vi "Replace -2 and -1.vi"(5 "Row  [ ] IN":T2, 9 "Table size":cluster{"# Column":u16, "# Row":u16}) -> (6 "Row  [ ] OUT":T2, 10 "Row and #colums [ ]":T1(array[cluster]))   [LabVIEW 2019, in "Exaprom PDF.lvlib"]
doc: "Version 1.1\nDeveloped by Jean-Marc Simard\nCopyright © 2012, Exaprom Inc.\nAll rights reserved.\nLicense: BSD\n\nWith iTextSharp 4.1.6 (http://itextsharp.sourceforge.net)\nunder Mozilla Public License Version 1.1\n(http://www.mozilla.org/MPL/MPL-1.1.html)"
uses:
  Controls/Table Controls/Table Appearance and Font Row [ ].ctl
  Controls/Table Controls/One Row Appearance.ctl
  Controls/Table Controls/Row from to.ctl
  Controls/Table Controls/Cell, Alignment, LS and Font - hide Vmerge.ctl
  Controls/Table Controls/Cell Type, Alignment and LS.ctl
  Controls/Table Controls/Cell Alignment 20px.ctl
  Controls/Table Controls/Text vertical arrangement.ctl
  Controls/Text Controls/Line spacing.ctl
  Controls/Table Controls/Cell Appearance.ctl
  Controls/Table Controls/Cell Border 20 px.ctl
  Controls/Table Controls/Merge Horizontal.ctl
  Controls/Table Controls/Merge Vertical.ctl
  Controls/Font Controls/Font complete cluster.ctl
  Controls/Font Controls/Font size.ctl
  Controls/Font Controls/Font color.ctl
  Controls/Font Controls/Type and encoding.ctl
  Controls/Text Controls/Unicode/Type and run direction.ctl
  Exaprom PDF.lvlib
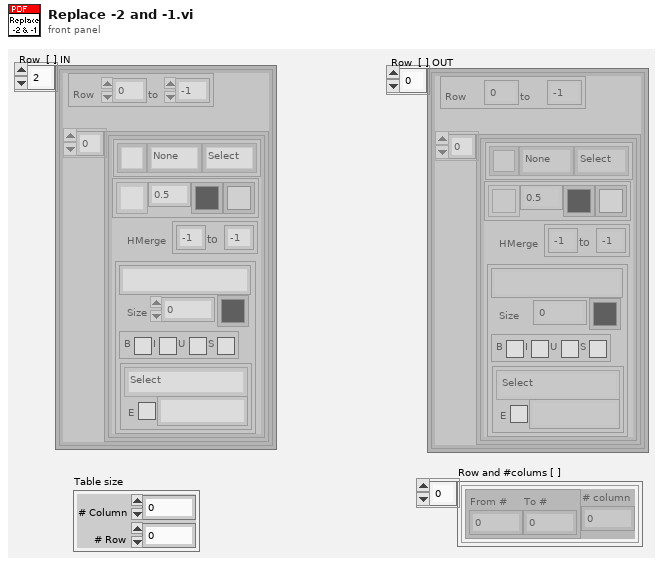
[diagram p1: front panel]
types:
  T1 = cluster{cluster{"From #":i16, "To #":i16}, "# column":u16}[]
  T2 = typedef "Exaprom PDF.lvlib/Table Appearance and Font Row [ ].ctl" = T3[]
  T3 = typedef "Exaprom PDF.lvlib/One Row Appearance.ctl" = cluster{"Row":T4, "Cell [ ]":T5[]}
  T4 = typedef "Exaprom PDF.lvlib/Row from to.ctl" = cluster{"From #":i16, "to #":i16}
  T5 = typedef "Exaprom PDF.lvlib/Cell, Alignment, LS and Font - hide Vmerge.ctl" = cluster{"Text":T6, "Cell Appearance":T10, "HMerge":T12, "VMerge":T13, "Font":T14}
  T6 = typedef "Exaprom PDF.lvlib/Cell Type, Alignment and LS.ctl" = cluster{"Cell Alignment":T7, "Text rotation":T8, "Line spacing":T9}
  T7 = typedef "Exaprom PDF.lvlib/Cell Alignment 20px.ctl" = u16
  T8 = typedef "Exaprom PDF.lvlib/Text vertical arrangement.ctl" = enum16{"None", "Clockwise", "Counterclockwise"}
  T9 = typedef "Exaprom PDF.lvlib/Line spacing.ctl" = enum16{"Select", "1.0", "1.5", "2.0"}
  T10 = typedef "Exaprom PDF.lvlib/Cell Appearance.ctl" = cluster{"Border":T11, "Thickness":sgl, "Color":u32, "BG":u32}
  T11 = typedef "Exaprom PDF.lvlib/Cell Border 20 px.ctl" = u16
  T12 = typedef "Exaprom PDF.lvlib/Merge Horizontal.ctl" = cluster{"From":i8, "to":i8}
  T13 = typedef "Exaprom PDF.lvlib/Merge Vertical.ctl" = cluster{"From":i8, "to":i8}
  T14 = typedef "Exaprom PDF.lvlib/Font complete cluster.ctl" = cluster{"Name":string, "Size":T15, "Color":T16, "Style":cluster{"Bold":bool, "Italic":bool, "Underline":bool, "Strikeout":bool}, "Type":T17}
  T15 = typedef "Exaprom PDF.lvlib/Font size.ctl" = sgl
  T16 = typedef "Exaprom PDF.lvlib/Font color.ctl" = u32
  T17 = typedef "Exaprom PDF.lvlib/Type and encoding.ctl" = cluster{"Type&direction":T18, "Embedded":bool, "Encoding":string}
  T18 = typedef "Exaprom PDF.lvlib/Type and run direction.ctl" = enum16{"Select", "ASCII", "UTF-16", "UTF-16 (default)", "UTF-16 (LTR)", "UTF-16 (RTL)"}
  T19 = cluster{cluster{"From #":i16, "From #":i16}, "Cell [ ]":T5[]}
  T20 = cluster{cluster{"From #":i16, "From #":i16}, u16}
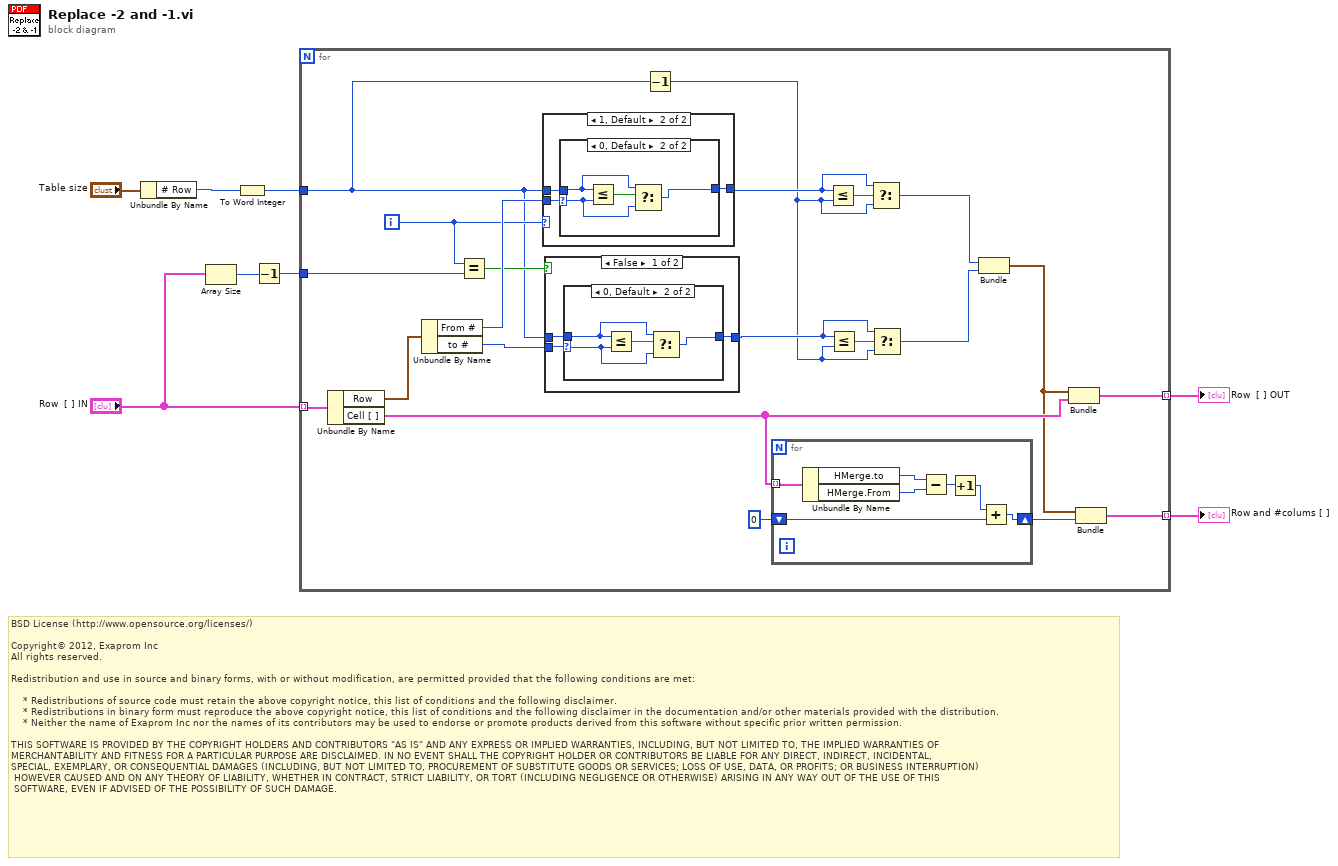
[diagram p0: block diagram]
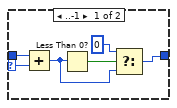
[diagram p2: hidden frame]
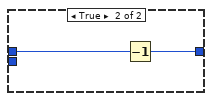
[diagram p3: hidden frame]
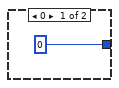
[diagram p4: hidden frame]
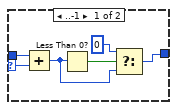
[diagram p5: hidden frame]
diagram:
  # "BSD License (http://www.opensource.org/licenses/)\n\nCopyright© 2012, Exaprom Inc\nAll rights reserved.\n\nRedistribution and use in source and binary forms, with or without modification, are permitted provided that the following conditions are met:\n\n    * Redistributions of source code must retain the above copyright notice, this list of conditions and the following disclaimer.\n    * Redistributions in binary form must reproduce the above copyright notice, this list of conditions and the following disclaimer in the documentation and/or other materials provided with the distribution.\n    * Neither the name of Exaprom Inc nor the names of its contributors may be used to endorse or promote products derived from this software without specific prior written permission.\n\nTHIS SOFTWARE IS PROVIDED BY THE COPYRIGHT HOLDERS AND CONTRIBUTORS \"AS IS\" AND ANY EXPRESS OR IMPLIED WARRANTIES, INCLUDING, BUT NOT LIMITED TO, THE IMPLIED WARRANTIES OF \nMERCHANTABILITY AND FITNESS FOR A PARTICULAR PURPOSE ARE DISCLAIMED. IN NO EVENT SHALL THE COPYRIGHT HOLDER OR CONTRIBUTORS BE LIABLE FOR ANY DIRECT, INDIRECT, INCIDENTAL,\nSPECIAL, EXEMPLARY, OR CONSEQUENTIAL DAMAGES (INCLUDING, BUT NOT LIMITED TO, PROCUREMENT OF SUBSTITUTE GOODS OR SERVICES; LOSS OF USE, DATA, OR PROFITS; OR BUSINESS INTERRUPTION)\n HOWEVER CAUSED AND ON ANY THEORY OF LIABILITY, WHETHER IN CONTRACT, STRICT LIABILITY, OR TORT (INCLUDING NEGLIGENCE OR OTHERWISE) ARISING IN ANY WAY OUT OF THE USE OF THIS\n SOFTWARE, EVEN IF ADVISED OF THE POSSIBILITY OF SUCH DAMAGE."
  n1 = Unbundle By Name("Table size") -> ("# Row"=w7:u16)
  n2 = Array Size(array="Row  [ ] IN") -> (size(s)=w4:i32)
  n3 = To Word Integer(number=w7) -> (16bit integer=w6:i16)
  n4 = Decrement(x=w4) -> (x-1=w3:i32)
  n5 = for {
    tunnel: "Row  [ ] IN" -> [w29] mode=indexing
    tunnel: w6 -> [w16]
    tunnel: [w27] -> w2 mode=indexing
    tunnel: w3 -> [w23]
    tunnel: [w17] -> w1 mode=indexing
    i -> [w24]
    n6 = Unbundle By Name(w29) -> ("Row"=w28:T4, "Cell [ ]"=w20:T5[])
    n7 = Unbundle By Name(w28) -> ("From #"=w26:i16, "to #"=w25:i16)
    n8 = Equal?(x=w24, y=w23) -> (x = y?=w22:bool)
    n9 = case shown="1, Default" w24 {
      tunnel: [i16 0 ("t") w55] -> w14
      tunnel: w16 -> [_ w54]
      tunnel: w26 -> [_ w53]
      frame 0 {
      }
      frame 1, Default {
        n10 = case shown="0, Default" w53 {
          selector: w53 -> [w56 w63]
          tunnel: [w61 w62] -> w55
          tunnel: w54 -> [w57 w64]
          frame ..-1 {
            n11 = Add(x=w57, y=w56) -> (x+y=w59:i16)
            n12 = Less Than 0?(x=w59) -> (x < 0?=w60:bool)
            n13 = Select(t=i16 0, s=w60, f=w59) -> (s? t:f=w61:i16)
          }
          frame 0, Default {
            n14 = Less Or Equal?(x=w64, y=w63) -> (x <= y?=w65:bool)
            n15 = Select(t=w64, s=w65, f=w63) -> (s? t:f=w62:i16)
          }
        }
      }
    }
    n16 = case shown="False" w22 {
      tunnel: w16 -> [w37 w50]
      tunnel: w25 -> [w38 _]
      tunnel: [w39 w51] -> w11
      frame False {
        n17 = case shown="0, Default" w38 {
          selector: w38 -> [w40 w47]
          tunnel: [w45 w46] -> w39
          tunnel: w37 -> [w41 w48]
          frame ..-1 {
            n18 = Add(x=w41, y=w40) -> (x+y=w43:i16)
            n19 = Less Than 0?(x=w43) -> (x < 0?=w44:bool)
            n20 = Select(t=i16 0, s=w44, f=w43) -> (s? t:f=w45:i16)
          }
          frame 0, Default {
            n21 = Less Or Equal?(x=w48, y=w47) -> (x <= y?=w49:bool)
            n22 = Select(t=w48, s=w49, f=w47) -> (s? t:f=w46:i16)
          }
        }
      }
      frame True {
        n23 = Decrement(x=w50) -> (x-1=w51:i16)
      }
    }
    n24 = Decrement(x=w16) -> (x-1=w10:i16)
    n25 = for {
      tunnel: w20 -> [w36] mode=indexing
      shift-right: [w31] -> w18
      shift-left: u16 0 -> [w30]
      n26 = Unbundle By Name(w36) -> ("HMerge.to"=w35:i8, "HMerge.From"=w33:i8)
      n27 = Subtract(x=w35, y=w33) -> (x-y=w34:i8)
      n28 = Increment(x=w34) -> (x+1=w32:i8)
      n29 = Add(x=w32, y=w30) -> (x+y=w31:u16)
    }
    n30 = Less Or Equal?(x=w14, y=w10) -> (x <= y?=w15:bool)
    n31 = Less Or Equal?(x=w11, y=w10) -> (x <= y?=w12:bool)
    n32 = Select(t=w14, s=w15, f=w10) -> (s? t:f=w13:i16)
    n33 = Select(t=w11, s=w12, f=w10) -> (s? t:f=w9:i16)
    n34 = Bundle("From #"=w13, "From #"=w9) -> (w19:cluster{"From #":i16, "From #":i16})  [unwired: 1 in]
    n35 = Bundle(w19, "Cell [ ]"=w20) -> (w27:T19)  [unwired: 1 in]
    n36 = Bundle(w19, w18) -> (w17:T20)  [unwired: 1 in]
  }
  "Row  [ ] OUT" <- w2
  "Row and #colums [ ]" <- w1
